vi "TransformToJointsOfSegment__slk_mt.vi"(8 "error in (no error)":errorcluster, 10 "joints[]":T1(array[cluster])) -> (0 "error out":errorcluster, 2 "joints[]":cluster{"X":i32, "Y":i32}[][](array[cluster]))   [LabVIEW 2013, in "Lazyboots Menu Tool.lvlib" / "Wire__slk_mt.lvclass"]
doc: "Transefers joints of wire {1D array} to the joints of segments {2D array}."
uses:
  Wire__slk_mt.lvclass
panel:
  # "TransformToJointsOfSegment__slk_mt.vi\nTransefers joints of wire {1D array} to the joints of segments {2D array}.\n\nNOTICE -- YOU MUST LEAVE THIS NOTICE IN PLACE.\n\nCopyright (c) 2011, LIANG LIU Shawn.Liu.cn@gmail.com\nAll rights reserved.\n\nRedistribution and use in source and binary forms, with or without modification, are permitted provided that the following conditions are met:\n-Redistributions of source code must retain the above copyright notice, this list of conditions and the following disclaimer.\n-Redistributions in binary form must reproduce the above copyright notice, this list of conditions and the following disclaimer in the documentation and/or other materials provided with the distribution.\n-Neither the name of the eLp nor the names of its contributors may be used to endorse or promote products derived from this software without specific prior written permission.\n\nTHIS SOFTWARE IS PROVIDED BY THE COPYRIGHT HOLDERS AND CONTRIBUTORS \"AS IS\" AND ANY EXPRESS OR IMPLIED WARRANTIES, INCLUDING, BUT NOT LIMITED TO, THE IMPLIED WARRANTIES OF MERCHANTABILITY AND FITNESS FOR A PARTICULAR PURPOSE ARE DISCLAIMED. IN NO EVENT SHALL THE COPYRIGHT HOLDER OR CONTRIBUTORS BE LIABLE FOR ANY DIRECT, INDIRECT, INCIDENTAL, SPECIAL, EXEMPLARY, OR CONSEQUENTIAL DAMAGES (INCLUDING, BUT NOT LIMITED TO, PROCUREMENT OF SUBSTITUTE GOODS OR SERVICES; LOSS OF USE, DATA, OR PROFITS; OR BUSINESS INTERRUPTION) HOWEVER CAUSED AND ON ANY THEORY OF LIABILITY, WHETHER IN CONTRACT, STRICT LIABILITY, OR TORT (INCLUDING NEGLIGENCE OR OTHERWISE) ARISING IN ANY WAY OUT OF THE USE OF THIS SOFTWARE, EVEN IF ADVISED OF THE POSSIBILITY OF SUCH DAMAGE."
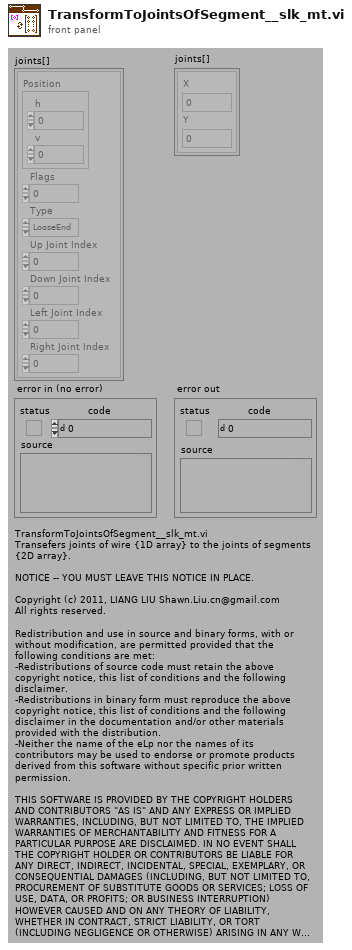
[diagram p1: front panel]
types:
  T1 = cluster{"Position":cluster{"h":i16, "v":i16}, "Flags":i32, "Type":enum32{"LooseEnd", "Endpoint", "Bend", "Junction"}, "Up Joint Index":i16, "Down Joint Index":i16, "Left Joint Index":i16, "Right Joint Index":i16}[]
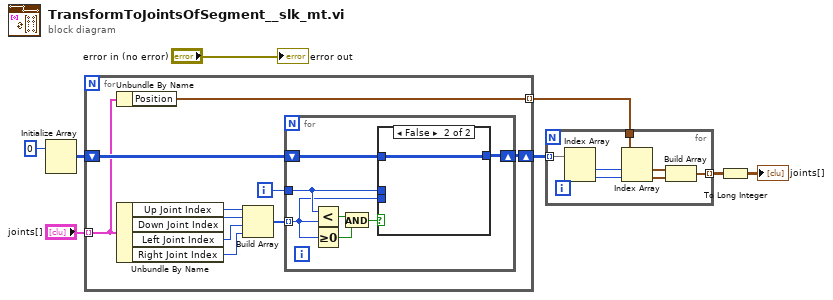
[diagram p0: block diagram]
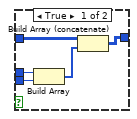
[diagram p2: hidden frame]
diagram:
  n1 = Initialize Array(0 ("dimension size")) -> (w7:i32[][])  [unwired: 2 out]
  n2 = for {
    tunnel: "joints[]" -> [w10] mode=indexing
    shift-right: [w12] -> w5
    shift-left: w7 -> [w13]
    tunnel: [w9] -> w4 mode=indexing
    i -> [w11]
    n3 = Unbundle By Name(w10) -> ("Position"=w9:cluster{"h":i16, "v":i16})
    n4 = Unbundle By Name(w10) -> ("Up Joint Index"=w18:i16, "Down Joint Index"=w17:i16, "Left Joint Index"=w16:i16, "Right Joint Index"=w15:i16)
    n5 = Build Array(w18, w17, w16, w15) -> (w14:i16[])
    n6 = for {
      tunnel: w14 -> [w19] mode=indexing
      shift-right: [w24] -> w12
      shift-left: w13 -> [w25]
      tunnel: w11 -> [w23]
      n7 = Less?(x=w23, y=w19) -> (x < y?=w22:bool)
      n8 = Greater Or Equal To 0?(x=w19) -> (x >= 0?=w21:bool)
      n9 = And(x=w22, y=w21) -> (x .and. y?=w20:bool)
      n10 = case shown="False" w20 {
        tunnel: w25 -> [w30 w31]
        tunnel: [w29 w31] -> w24
        tunnel: w23 -> [w28 _]
        tunnel: w19 -> [w26 _]
        frame True {
          n11 = Build Array(w28, w26) -> (w27:i32[])
          n12 = Build Array (concatenate)(w30, w27) -> (w29:i32[][])
        }
        frame False {
        }
      }
    }
  }
  n13 = for {
    tunnel: w5 -> [w38] mode=indexing
    tunnel: w4 -> [w35]
    tunnel: [w32] -> w3 mode=indexing
    n14 = Index Array(array=w38) -> (element #1=w37:i32, element #2=w36:i32)  [unwired: 2 in]
    n15 = Index Array(array=w35, index #1=w37, index #2=w36) -> (element #1=w34:cluster{"h":i16, "v":i16}, element #2=w33:cluster{"h":i16, "v":i16})
    n16 = Build Array(w34, w33) -> (w32:cluster{"h":i16, "v":i16}[])
  }
  n17 = To Long Integer(number=w3) -> (32bit integer=→"joints[]":cluster{"h":i32, "v":i32}[][])
  "error out" <- "error in (no error)"
